vi "Save Raw FGV.vi"(6 "Save Options":enum16{"Save  Raw", "Fetch Raw", "Error"}(ring), 8 "error in (no error)":errorcluster, 10 "Data Cluster":T1, 11 "Image In":T2) -> (0 "error out":errorcluster, 2 "File Name":path, 3 "Image":T2(plugin-control))   [LabVIEW 2021]
uses:
  <vilib>/vision/Image Controls.llb/IMAQ Image.ctl
  <userlib>/_MGI/Error Reporter/MGI Error Reporter Base/MGI Error Reporter Base.lvclass
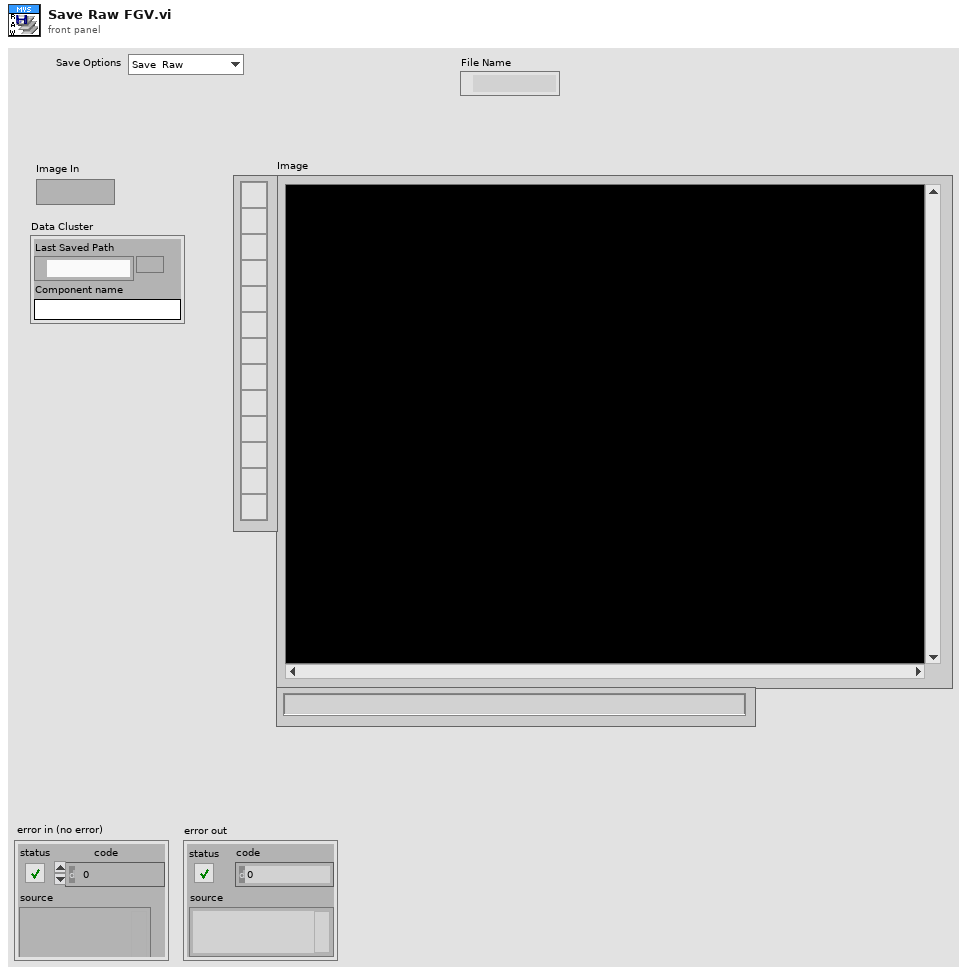
[diagram p1: front panel]
types:
  T1 = cluster{"Last Saved Path":path, "Component name":string}
  T2 = typedef "IMAQ Image.ctl" = refnum<image>
  T3 = typedef "Image Type" = u32
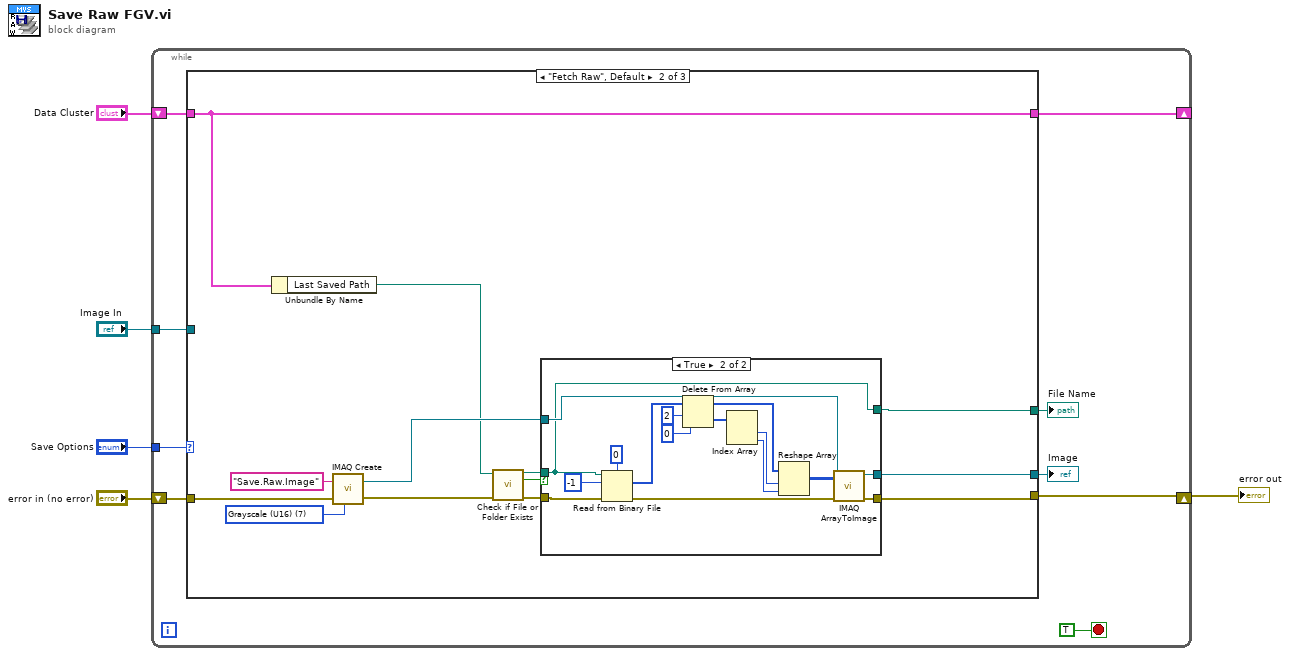
[diagram p0: block diagram]
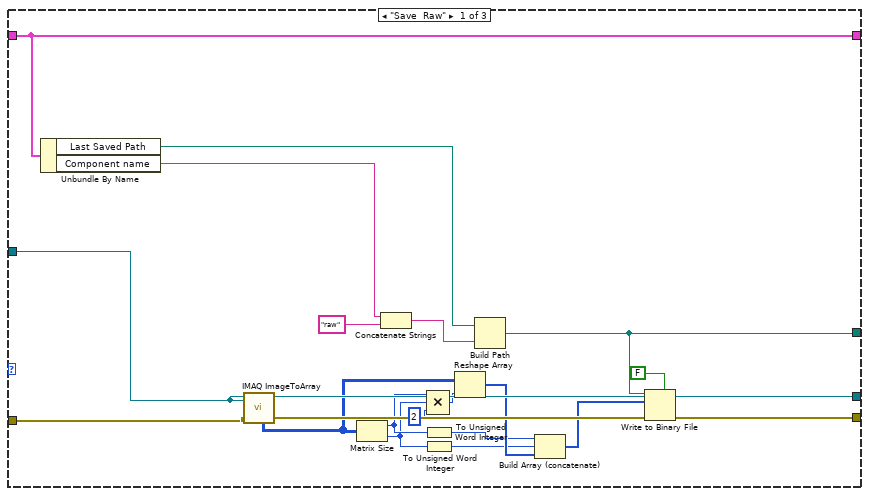
[diagram p2: hidden frame]
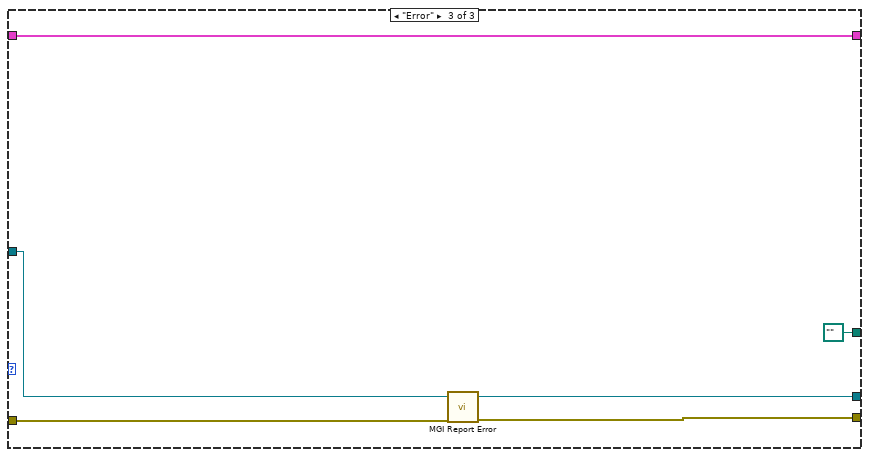
[diagram p4: hidden frame]
diagram:
  n1 = while {
    tunnel: "Save Options" -> [w13]
    shift-right: [w10] -> _
    shift-left: "Data Cluster" -> [w11]
    tunnel: "Image In" -> [w7]
    shift-right: [w14] -> w5
    shift-left: "error in (no error)" -> [w12]
    stop <- TRUE stop-if-true
    n2 = case shown="\"Fetch Raw\", Default" w13 {
      tunnel: [w33 w42 w71] -> w14
      tunnel: w12 -> [w26 w41 w70]
      tunnel: [w34 w47 w69] -> w10
      tunnel: w11 -> [w34 w47 w69]
      tunnel: [w27 w43 w68] -> w8
      tunnel: w7 -> [w27 _ w68]
      tunnel: [w15 w35 path "" ("dup path")] -> w6
      frame "Save  Raw" {
        n3 = Unbundle By Name(w34) -> ("Last Saved Path"=w32:path, "Component name"=w28:string)
        n4 = call "IMAQ ImageToArray"("error in (no error)"=w26, "Image"=w27) -> ("Image Pixels (U16)"=w25:u16[][], "error out"=w29:errorcluster)  [unwired: 2 in, 3 out]
        n5 = Matrix Size(0:w25) -> (1:w21:i32, 2:w20:i32)
        n6 = Concatenate Strings(w28, "raw" ("string")) -> (w31:string)
        n7 = To Unsigned Word Integer(number=w21) -> (unsigned 16bit integer=w17:u16)
        n8 = To Unsigned Word Integer(number=w20) -> (unsigned 16bit integer=w16:u16)
        n9 = Compound Arithmetic op=MULTIPLY(w21, w20, 2 ("value")) -> (w23:i32)
        n10 = Reshape Array(w25, w23) -> (w19:u16[])
        n11 = Build Path(base path=w32, name or relative path=w31) -> (appended path=w15:path)
        n12 = Build Array (concatenate)(w17, w16, w19) -> (w18:u16[])
        n13 = Write to Binary File(file (use dialog)=w15, data=w18, error in=w29, 5:FALSE ("prepend array or string size? (T)")) -> (error out=w33:errorcluster)  [unwired: 2 in, 2 out]
      }
      frame "Fetch Raw", Default {
        w39 = T3 7 items=["Grayscale (U8)", "Grayscale (I16)", "Grayscale (SGL)", "Complex (CSG)", "RGB (U32)", "HSL (U32)", "RGB (U64)", "Grayscale (U16)"] ("Image Type")
        n14 = Unbundle By Name(w47) -> ("Last Saved Path"=w36:path)
        n15 = call "IMAQ Create"("Image Name"="Save.Raw.Image", "Image Type"=w39, "error in (no error)"=w41) -> ("New Image"=w37:T2, "error out"=w40:errorcluster)  [unwired: 2 in]
        n16 = call <vilib>:"Check if File or Folder Exists.vi"("error in (no error)"=w40, "path"=w36) -> ("error out"=w46:errorcluster, "file or folder exists?"=w45:bool, "dup path"=w44:path)  [unwired: 7 in]
        n17 = case shown="True" w45 {
          tunnel: [w50 w54] -> w42
          tunnel: w46 -> [w50 w57]
          tunnel: w44 -> [w48 w51]
          tunnel: [w49 w55] -> w43
          tunnel: w37 -> [w49 w52]
          tunnel: [w48 w51] -> w35
          frame False {
          }
          frame True {
            n18 = Read from Binary File(5:u16 0, 8:w57, 10:-1 ("count (1)"), 11:w51) -> (0:w56:errorcluster, 2:w64:u16[])  [unwired: 2 in, 2 out]
            n19 = Delete From Array(array=w64, length=2, index=0) -> (deleted portion=w61:u16[], array with subset deleted=w58:u16[])
            n20 = Index Array(array=w61) -> (element #1=w60:u16, element #2=w59:u16)  [unwired: 2 in]
            n21 = Reshape Array(w58, w60, w59) -> (w53:u16[][])
            n22 = call "IMAQ ArrayToImage"("Image Pixels (U16)"=w53, "error in (no error)"=w56, "Image"=w52) -> ("error out"=w54:errorcluster, "Image Out"=w55:T2)  [unwired: 7 in]
          }
        }
      }
      frame "Error" {
        n23 = call <userlib>:"MGI Report Error.vi"("error in"=w70) -> ("no error"=w71:errorcluster)  [unwired: 10 in]
      }
    }
    "Image" <- w8
    "File Name" <- w6
  }
  "error out" <- w5
